vi "Cannon Cannon.vi"(1 "Cannon Info In":T2) -> (0 "Cannon Info Out?":T2)   [LabVIEW 2013]
uses:
  <vilib>/Rock Robotics/WPI/Solenoid/WPI_SolenoidValue.ctl
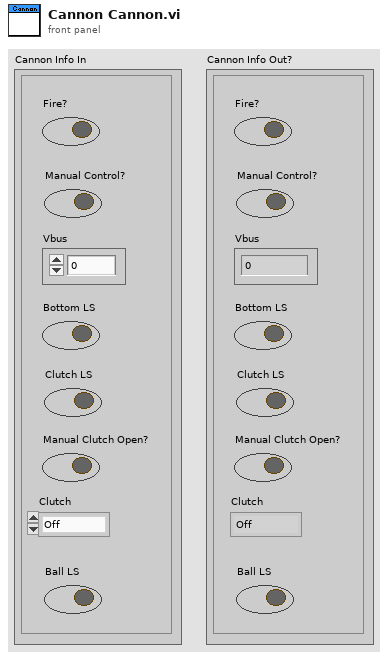
[diagram p1: front panel]
types:
  T1 = typedef "WPI_SolenoidValue.ctl" = enum16{"Off", "On", "Forward", "Reverse"}
  T2 = cluster{"Fire?":bool, "Manual Control?":bool, "Vbus":dbl, "Bottom LS":bool, "Clutch LS ":bool, "Manual Clutch Open?":bool, "Clutch":T1, "Ball LS":bool}
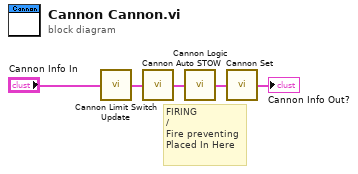
[diagram p0: block diagram]
diagram:
  # "FIRING\n/ \nFire preventing\nPlaced In Here"
  n1 = call "Cannon Limit Switch Update.vi"("Cannon Info In"="Cannon Info In") -> ("Cannon Info Out?"=w1:T2)
  n2 = call "Cannon Auto STOW.vi"("Cannon Info In"=w1) -> ("Cannon Info Out?"=w2:T2)
  n3 = call "Cannon Logic.vi"("Cannon Info In"=w2) -> ("Cannon Info Out?"=w3:T2)
  n4 = call "Cannon Set.vi"("Cannon Info In"=w3) -> ("Cannon Info Out?"=→"Cannon Info Out?":T2)
